vi "ex_4_6.vi"() -> ()   [LabVIEW 2020]
uses:
  <vilib>/numeric/Random Number (Range) U64.vi
  <vilib>/numeric/sub_Random U32.vi
panel:
  out "Multiplied Array":u64[](array[numeric])
  out "Random Numbers Array":u64[](array[numeric])
  in  "Elements Number":i32
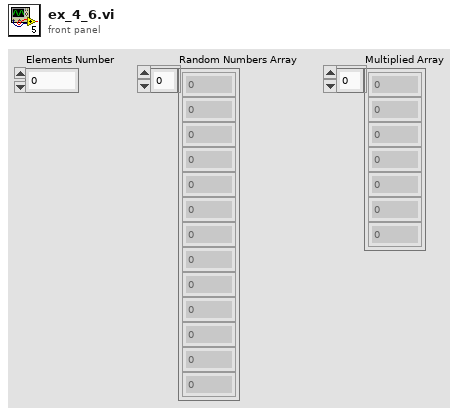
[diagram p1: front panel]
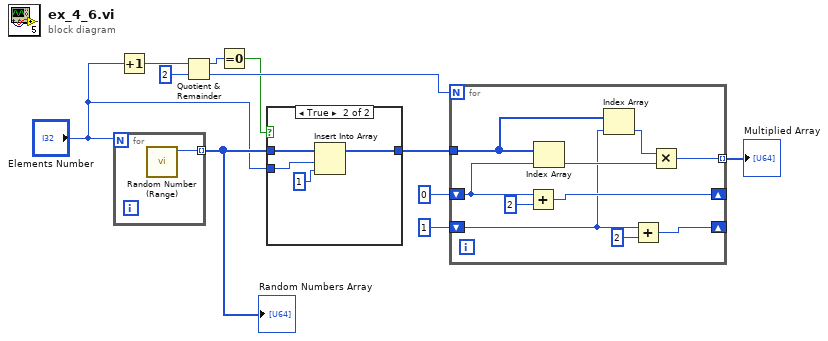
[diagram p0: block diagram]
diagram:
  n1 = for {
    N: "Elements Number" -> [_]
    tunnel: [w12] -> w3 mode=indexing
    n2 = call-poly <vilib>:"Random Number (Range).vi"() -> ("number"=w12:u64)  [unwired: 11 in]
  }
  "Random Numbers Array" <- w3
  n3 = Increment(x="Elements Number") -> (x+1=w11:i32)
  n4 = Quotient & Remainder(x=w11, y=2) -> (x-y*floor(x/y)=w5:i32, floor(x/y)=w9:i32)
  n5 = Equal To 0?(x=w5) -> (x = 0?=w4:bool)
  n6 = case shown="True" w4 {
    tunnel: w3 -> [w13 w17]
    tunnel: [w13 w16] -> w2
    tunnel: "Elements Number" -> [_ w14]
    frame False {
    }
    frame True {
      n7 = Insert Into Array(array=w17, index=w14, new element=u64 1 ("new element/subarray")) -> (w16:u64[])
    }
  }
  n8 = for {
    N: w9 -> [_]
    tunnel: w2 -> [w22]
    shift-right: [w26] -> _
    shift-left: 0 -> [w27]
    shift-right: [w23] -> _
    shift-left: 1 -> [w18]
    tunnel: [w19] -> w6 mode=indexing
    n9 = Add(x=w27, y=2) -> (x+y=w26:i32)
    n10 = Index Array(array=w22, index=w27) -> (element=w20:u64)
    n11 = Index Array(array=w22, index=w18) -> (element=w21:u64)
    n12 = Add(x=w18, y=2) -> (x+y=w23:i32)
    n13 = Multiply(x=w21, y=w20) -> (x*y=w19:u64)
  }
  "Multiplied Array" <- w6
